vi "addSkipped.vi"(8 "error in (no error)":errorcluster, 10 "test":refnum<class>, 11 "TestTestResult in":refnum<class "_TextTestResult.lvclass">) -> (0 "error out":errorcluster, 3 "TestTestResult out":refnum<class "_TextTestResult.lvclass">)   [LabVIEW 2011, in "_TextTestResult.lvclass"]
uses:
  _TextTestResult.lvclass
  TestCase/TestCase.lvclass
  TestResult/TestResult.lvclass
  _TextTestResult.lvclass/_TextTestResult.ctl
panel:
  # "JKI VI Tester for LabVIEW\nhttp://jkisoft.com/vi-tester\nCopyright (C) 2007-2009, JKI <info@jkisoft.com>\nALL RIGHTS RESERVED"
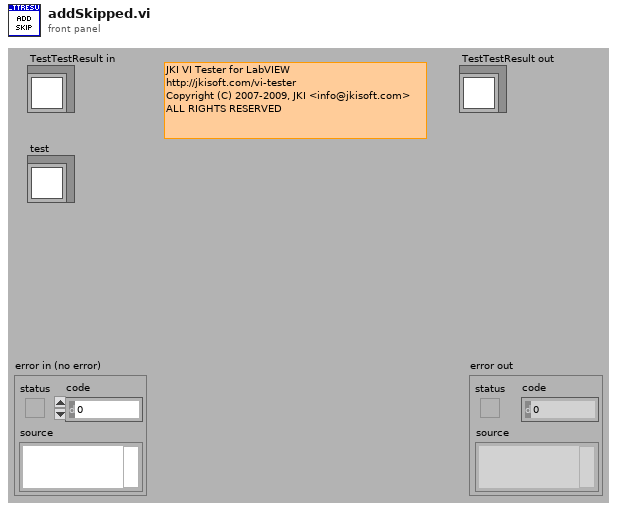
[diagram p1: front panel]
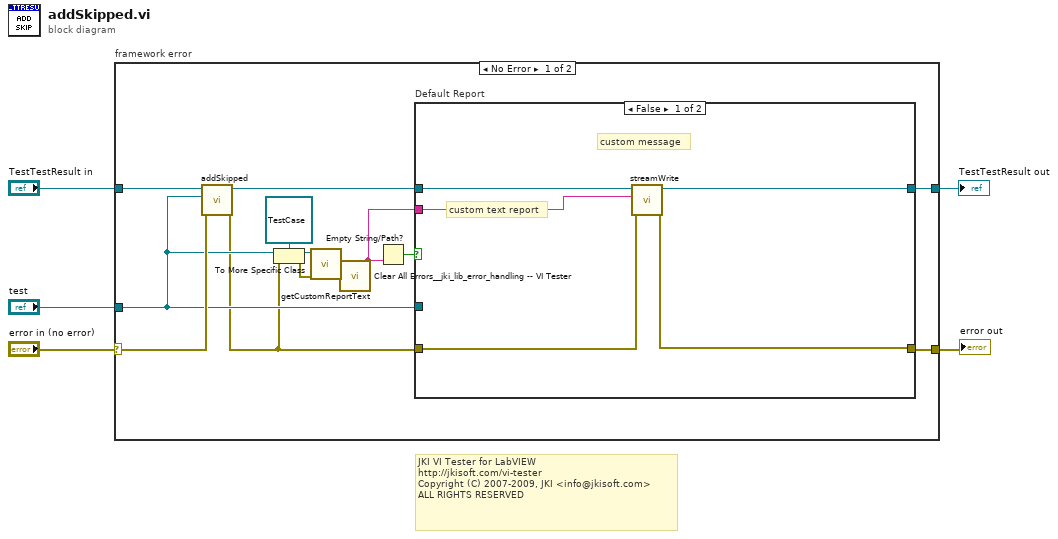
[diagram p0: block diagram]
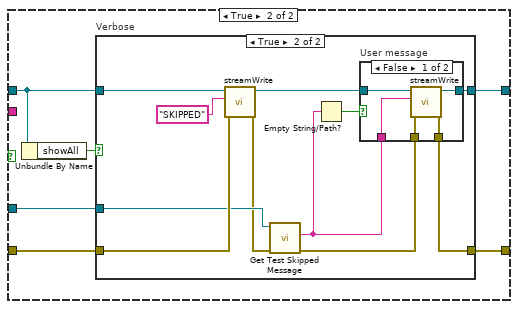
[diagram p2: hidden frame]
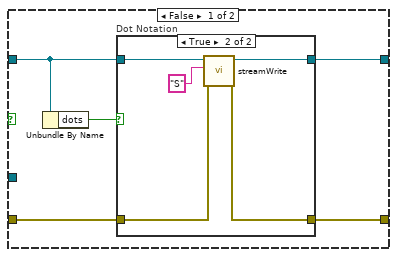
[diagram p3: hidden frame]
diagram:
  # "JKI VI Tester for LabVIEW\nhttp://jkisoft.com/vi-tester\nCopyright (C) 2007-2009, JKI <info@jkisoft.com>\nALL RIGHTS RESERVED"
  n1 = case "framework error" shown="No Error" "error in (no error)" {
    selector: "error in (no error)" -> [w17 w61]
    tunnel: [w15 w61] -> w4
    tunnel: [w16 w60] -> w2
    tunnel: "TestTestResult in" -> [w18 w60]
    tunnel: "test" -> [w9 _]
    frame No Error {
      n2 = call-parent "addSkipped.vi"("error in (no error)"=w17, "test"=w9, "TestResult in"=w18) -> ("error out"=w8:errorcluster, "TestResult out"=w14:refnum<class "_TextTestResult.lvclass">)  [unwired: 7 in]
      n3 = To More Specific Class(target class=refnum<class "TestCase.lvclass"> refnum ("TestCase in"), reference=w9, error in=w8) -> (specific class reference=w11:refnum<class "TestCase.lvclass">, error out=w13:errorcluster)
      n4 = call-dynamic "getCustomReportText.vi"("error in (no error)"=w13, "TestCase in"=w11) -> ("error out"=w10:errorcluster, "customReportText"=w6:string)  [unwired: 7 in, 1 out]
      n5 = call "Clear All Errors__jki_lib_error_handling -- VI Tester.vi"("error in"=w10) -> ()  [unwired: 4 in, 1 out]
      n6 = Empty String/Path?(string/path=w6) -> (empty?=w7:bool)
      n7 = case "Default Report" shown="False" w7 {
        tunnel: [w22 w29] -> w16
        tunnel: [w20 w28] -> w15
        tunnel: w14 -> [w23 w26]
        tunnel: w9 -> [_ w25]
        tunnel: w8 -> [w21 w24]
        tunnel: w6 -> [w19 _]
        frame False {
          # "custom text report"
          # "custom message"
          n8 = call "streamWrite.vi"("error in (no error)"=w21, "String"=w19, "TestTestResult in"=w23) -> ("error out"=w20:errorcluster, "TestTestResult out"=w22:refnum<class "_TextTestResult.lvclass">)  [unwired: 7 in]
        }
        frame True {
          n9 = Unbundle By Name(w26) -> ("showAll"=w27:bool)
          n10 = case "Verbose" shown="True" w27 {
            tunnel: w26 -> [w33 w52]
            tunnel: w24 -> [w31 w50]
            tunnel: [w30 w44] -> w28
            tunnel: [w34 w47] -> w29
            tunnel: w25 -> [_ w49]
            frame False {
              n11 = Unbundle By Name(w33) -> ("dots"=w32:bool)
              n12 = case "Dot Notation" shown="True" w32 {
                tunnel: w33 -> [w35 w41]
                tunnel: w31 -> [w36 w38]
                tunnel: [w36 w37] -> w30
                tunnel: [w35 w40] -> w34
                frame False {
                }
                frame True {
                  n13 = call "streamWrite.vi"("error in (no error)"=w38, "String"="S" ("element"), "TestTestResult in"=w41) -> ("error out"=w37:errorcluster, "TestTestResult out"=w40:refnum<class "_TextTestResult.lvclass">)  [unwired: 7 in]
                }
              }
            }
            frame True {
              n14 = call "streamWrite.vi"("error in (no error)"=w50, "String"="SKIPPED" ("element"), "TestTestResult in"=w52) -> ("error out"=w45:errorcluster, "TestTestResult out"=w48:refnum<class "_TextTestResult.lvclass">)  [unwired: 7 in]
              n15 = call "Get Test Skipped Message.vi"("error in"=w45, "Test In"=w49) -> ("error out"=w46:errorcluster, "skipMessage"=w43:string)  [unwired: 6 in, 2 out]
              n16 = Empty String/Path?(string/path=w43) -> (empty?=w42:bool)
              n17 = case "User message" shown="False" w42 {
                tunnel: w48 -> [w57 w59]
                tunnel: [w56 w59] -> w47
                tunnel: w46 -> [w55 w58]
                tunnel: [w54 w58] -> w44
                tunnel: w43 -> [w53 _]
                frame False {
                  n18 = call "streamWrite.vi"("error in (no error)"=w55, "String"=w53, "TestTestResult in"=w57) -> ("error out"=w54:errorcluster, "TestTestResult out"=w56:refnum<class "_TextTestResult.lvclass">)  [unwired: 7 in]
                }
                frame True {
                }
              }
            }
          }
        }
      }
    }
    frame Error {
    }
  }
  "error out" <- w4
  "TestTestResult out" <- w2
